vi "Stop Core.vi"(10 "final error code":i32, 11 "BuildServer in":refnum<class "BuildServer.lvclass">) -> (3 "BuildServer out":refnum<class "BuildServer.lvclass">)   [LabVIEW 2017, in "BuildServer.lvlib" / "BuildServer.lvclass"]
doc: "(<B>Filename</B>: Actor Framework.lvlib:Actor.lvclass:Stop Core.vi)\n\nDefines what the actor does before it stops. Use the <B>final error code</B> input to determine whether the actor shut down in response to an error.\n\nBy default, this method does nothing. A descendant class may override it to define behavior, such as shutting down any processes the actor initiated in its override of the Actor Core method."
uses:
  BuildServer.lvclass
  <vilib>/ActorFramework/Stop Msg/Stop Msg.lvclass
  <vilib>/Ekim/LUT/LUT/LUT.lvclass
  WebSocket Server/Actors/Actor wHelper/Actor wHelper/Actor wHelper.lvclass
  Classes/Comm Interface/Comm Interface.lvclass
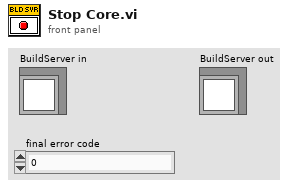
[diagram p1: front panel]
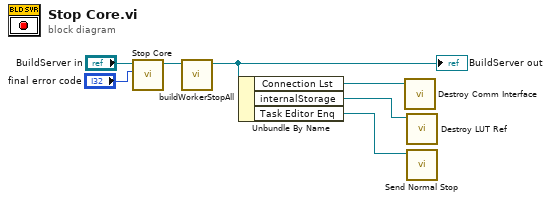
[diagram p0: block diagram]
diagram:
  n1 = call-parent "Stop Core.vi"("final error code"="final error code", "Actor wHelper in"="BuildServer in") -> ("Actor wHelper out"=w3:refnum<class "BuildServer.lvclass">)  [unwired: 9 in]
  n2 = call "buildWorkerStopAll.vi"("BuildServer in"=w3) -> ("BuildServer out"=w2:refnum<class "BuildServer.lvclass">)  [unwired: 9 in, 1 out]
  "BuildServer out" <- w2
  n3 = Unbundle By Name(w2) -> ("Connection Lst"=w1:refnum<class "Comm Interface.lvclass">, "internalStorage"=w5:refnum<class "LUT.lvclass">, "Task Editor Enq"=w4:refnum<class "Message Enqueuer.lvclass">)
  n4 = call "Destroy Comm Interface.vi"("Comm Interface in"=w1) -> ()  [unwired: 9 in, 2 out]
  n5 = call <vilib>:"Destroy LUT Ref.vi"("LUT in"=w5) -> ()  [unwired: 10 in, 1 out]
  n6 = call <vilib>:"Send Normal Stop.vi"("Message Enqueuer"=w4) -> ()  [unwired: 10 in, 1 out]
